vi "AlGaInPAs_Layer.vi"(2 "Debug Mode":bool, 3 "Elapsed Time (s)":dbl, 4 "State":enum16{"Edit", "Start", "Run", "End", "Idle"}(ring), 5 "Argument List In":string[](array[string])) -> (0 "Status Out":string, 1 "Argument List Out":string[](array[string]))   [LabVIEW 2011]
panel:
  out "Status Out 6":string
  out "Status Out 5":string
  out "Status Out 4":string
  out "Status Out 3":string
  out "In?":bool
  out "Ga?":bool
  out "Al?":bool
  out "AsH3?":bool
  out "PH3?":bool
  out "Status Out 2":string
  in  "AsH3 Flow":dbl
  in  "AsH3 run":bool
  in  "Al_run":bool
  in  "Al Flow":dbl
  in  "PH3 run":bool
  in  "In run":bool
  in  "Ga run":bool
  in  "PH3 Flow":dbl
  in  "In Flow":dbl
  in  "Ga Flow":dbl
  in  "Cancel":bool
  in  "OK":bool
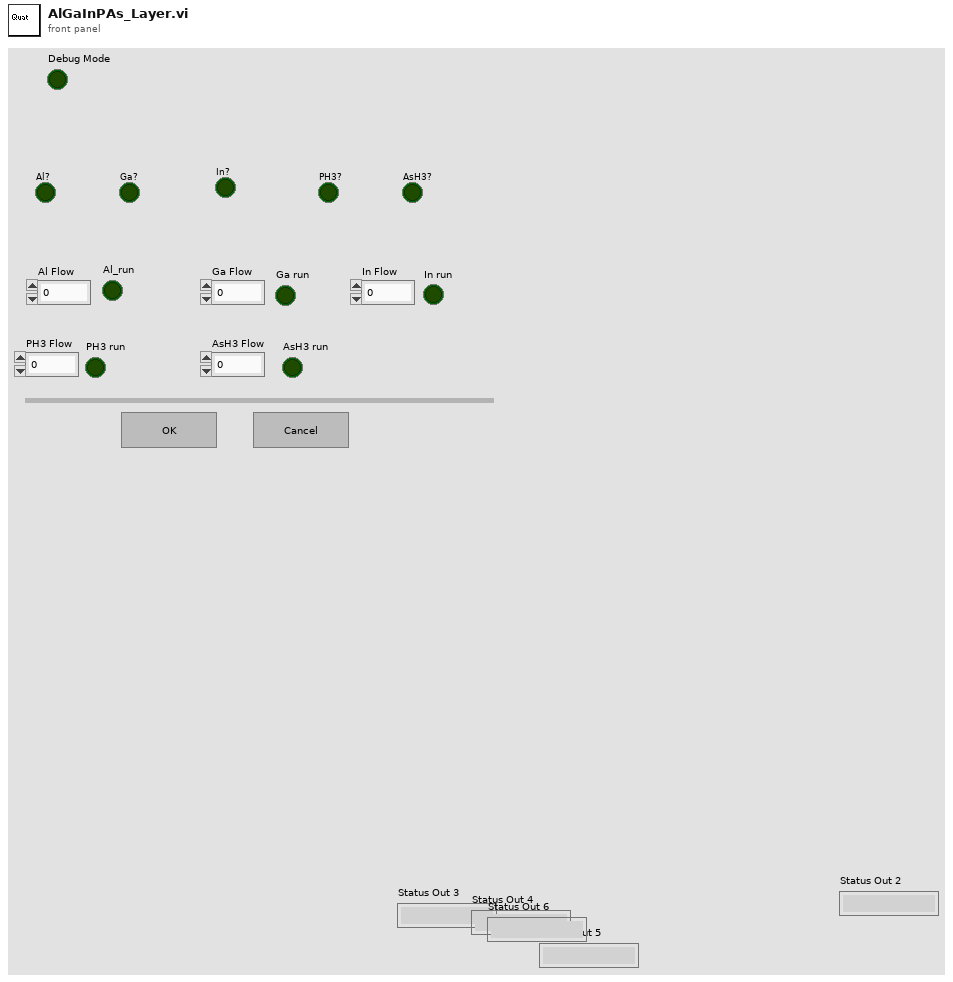
[diagram p1: front panel]
types:
  T1 = enum16{"Discrete", "Continuous", "Instantaneous"}
  T2 = enum32{"Invalid", "Default", "Floating", "Floating/Auto-Hide", "Modal"}
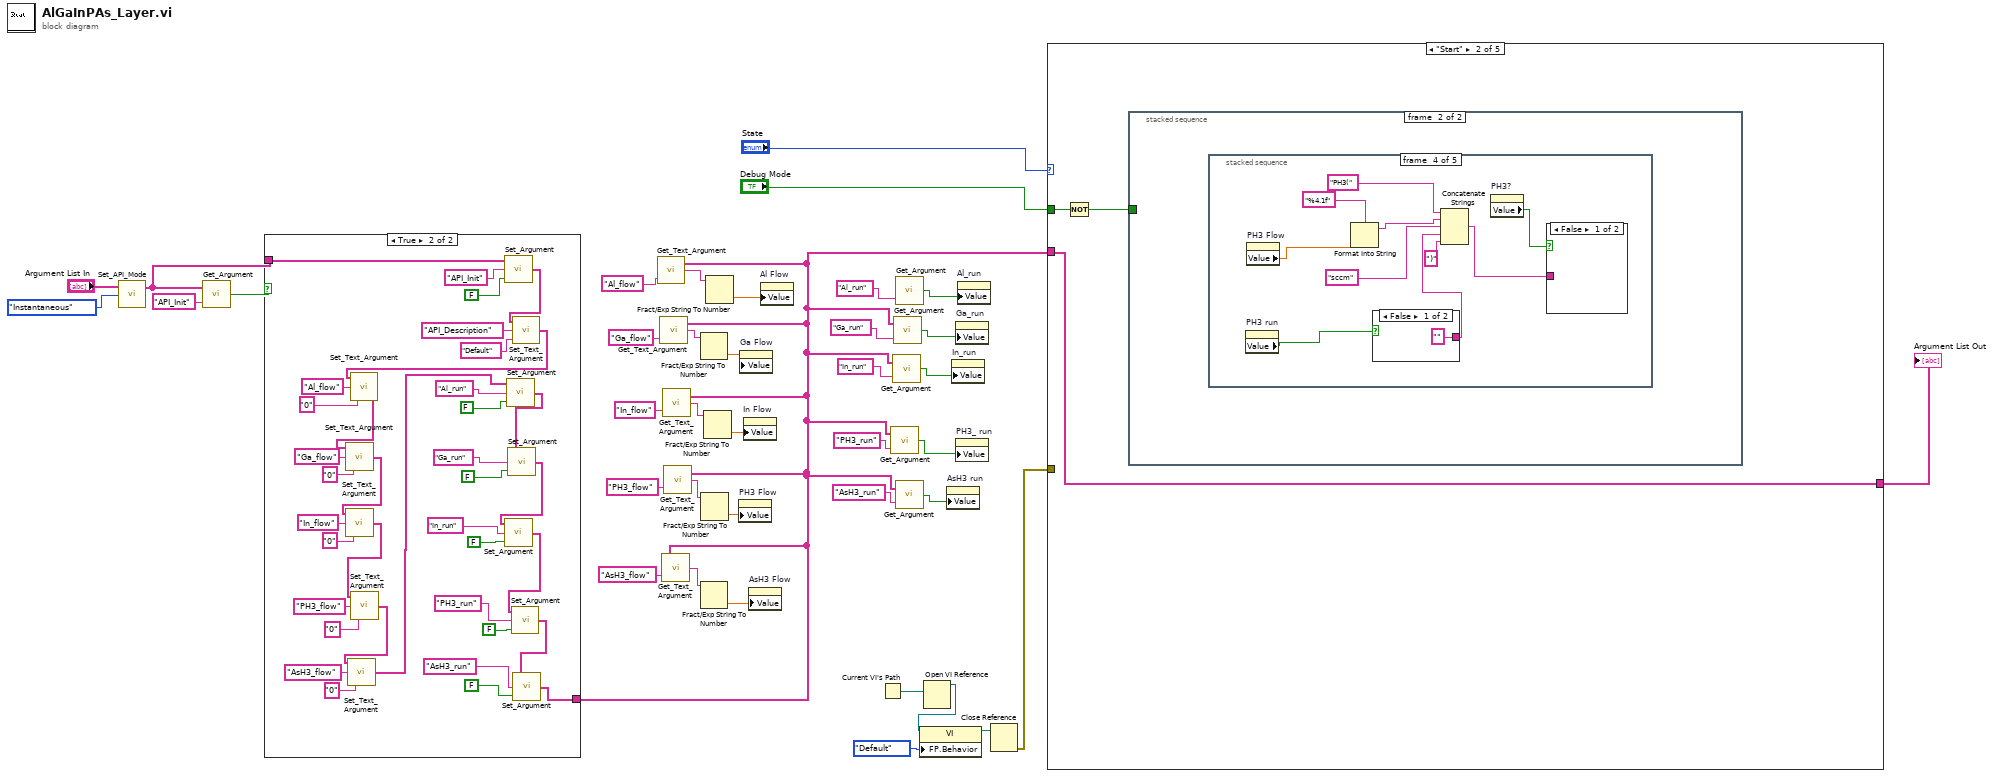
[diagram p0: block diagram]
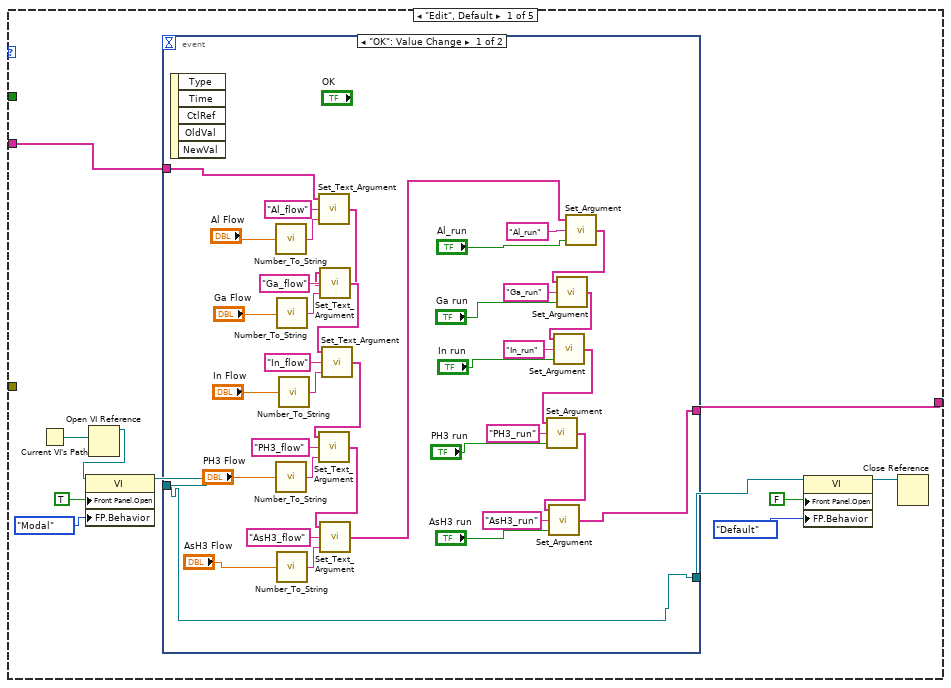
[diagram p3: hidden frame]
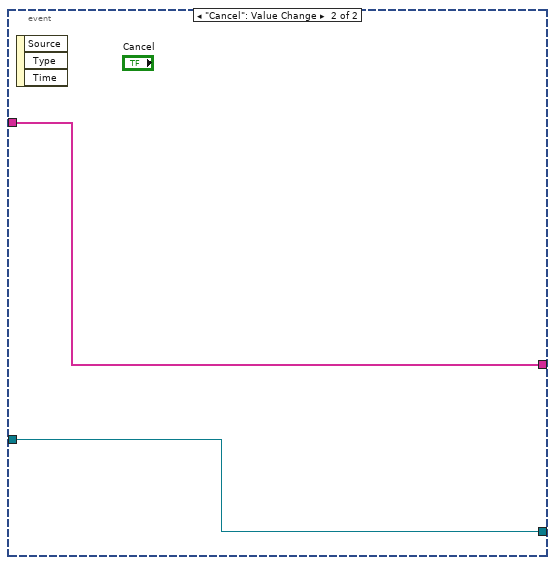
[diagram p4: hidden frame]
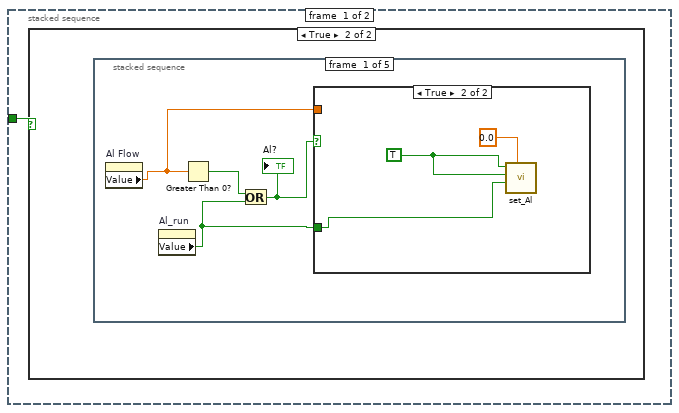
[diagram p5: hidden frame]
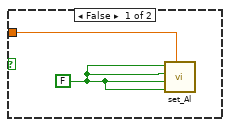
[diagram p7: hidden frame]
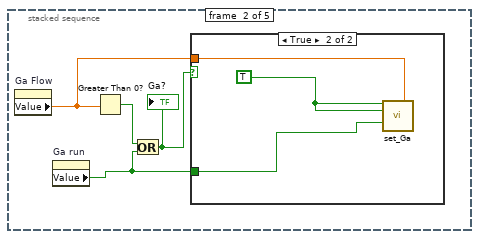
[diagram p8: hidden frame]
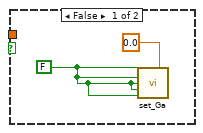
[diagram p9: hidden frame]
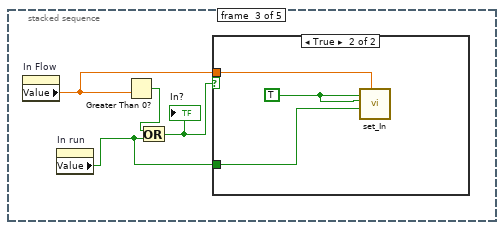
[diagram p10: hidden frame]
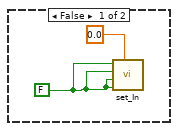
[diagram p11: hidden frame]
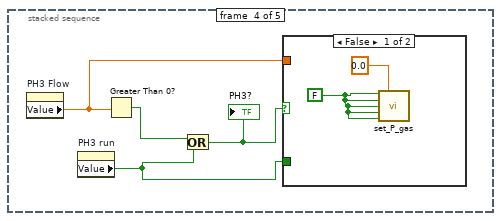
[diagram p12: hidden frame]
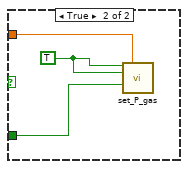
[diagram p13: hidden frame]
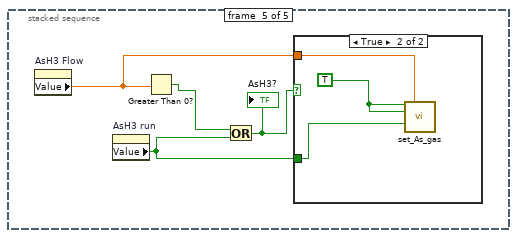
[diagram p14: hidden frame]
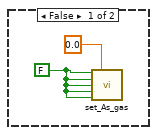
[diagram p15: hidden frame]
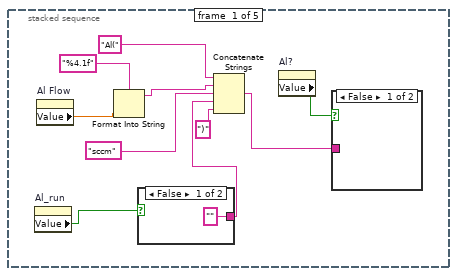
[diagram p16: hidden frame]
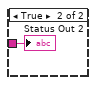
[diagram p17: hidden frame]
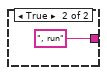
[diagram p18: hidden frame]
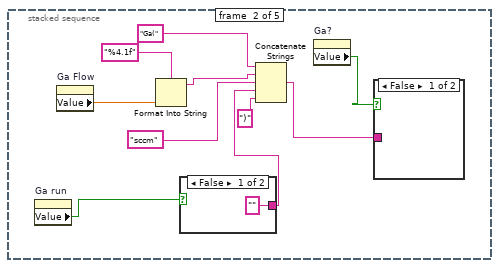
[diagram p19: hidden frame]
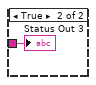
[diagram p20: hidden frame]
diagram:
  n1 = call "Set_API_Mode.vi"("API Mode"=T1."Instantaneous", "Argument List In"="Argument List In") -> ("Argument List Out"=w26:string[])  [unwired: 2 out]
  n2 = call "Get_Argument.vi"("Argument"="API_Init", "Argument List"=w26) -> ("Enabled"=w27:bool)
  n3 = case shown="True" w27 {
    tunnel: w26 -> [w40 w77]
    tunnel: [w40 w53] -> w5
    frame False {
    }
    frame True {
      n4 = call "Set_Argument.vi"("Enable"=FALSE, "Argument"="API_Init", "Argument List In"=w77) -> ("Argument List Out"=w74:string[])
      n5 = call "Set_Text_Argument.vi"("Text"="Default", "Argument"="API_Description", "Argument List In"=w74) -> ("Argument List Out"=w45:string[])
      n6 = call "Set_Text_Argument.vi"("Text"="0", "Argument"="Al_flow", "Argument List In"=w45) -> ("Argument List Out"=w44:string[])
      n7 = call "Set_Text_Argument.vi"("Text"="0", "Argument"="Ga_flow", "Argument List In"=w44) -> ("Argument List Out"=w67:string[])
      n8 = call "Set_Text_Argument.vi"("Text"="0", "Argument"="In_flow", "Argument List In"=w67) -> ("Argument List Out"=w43:string[])
      n9 = call "Set_Text_Argument.vi"("Text"="0", "Argument"="PH3_flow", "Argument List In"=w43) -> ("Argument List Out"=w55:string[])
      n10 = call "Set_Text_Argument.vi"("Text"="0", "Argument"="AsH3_flow", "Argument List In"=w55) -> ("Argument List Out"=w42:string[])
      n11 = call "Set_Argument.vi"("Enable"=FALSE, "Argument"="Al_run", "Argument List In"=w42) -> ("Argument List Out"=w48:string[])
      n12 = call "Set_Argument.vi"("Enable"=FALSE, "Argument"="Ga_run", "Argument List In"=w48) -> ("Argument List Out"=w58:string[])
      n13 = call "Set_Argument.vi"("Enable"=FALSE, "Argument"="In_run", "Argument List In"=w58) -> ("Argument List Out"=w41:string[])
      n14 = call "Set_Argument.vi"("Enable"=FALSE, "Argument"="PH3_run", "Argument List In"=w41) -> ("Argument List Out"=w51:string[])
      n15 = call "Set_Argument.vi"("Enable"=FALSE, "Argument"="AsH3_run", "Argument List In"=w51) -> ("Argument List Out"=w53:string[])
    }
  }
  n16 = call "Get_Text_Argument.vi"("Argument"="Al_flow", "Argument List"=w5) -> ("Text"=w6:string)
  n17 = call "Get_Text_Argument.vi"("Argument"="Ga_flow", "Argument List"=w5) -> ("Text"=w22:string)
  n18 = call "Get_Text_Argument.vi"("Argument"="AsH3_flow", "Argument List"=w5) -> ("Text"=w18:string)
  n19 = call "Get_Text_Argument.vi"("Argument"="In_flow", "Argument List"=w5) -> ("Text"=w20:string)
  n20 = call "Get_Text_Argument.vi"("Argument"="PH3_flow", "Argument List"=w5) -> ("Text"=w17:string)
  n21 = Fract/Exp String To Number(string=w22) -> (number=w21:dbl)  [unwired: 4 out]
  n22 = Fract/Exp String To Number(string=w18) -> (number=w1:dbl)  [unwired: 4 out]
  n23 = Fract/Exp String To Number(string=w17) -> (number=w16:dbl)  [unwired: 4 out]
  n24 = Fract/Exp String To Number(string=w20) -> (number=w19:dbl)  [unwired: 4 out]
  n25 = Fract/Exp String To Number(string=w6) -> (number=w2:dbl)  [unwired: 4 out]
  n26 = property on="PH3 Flow" class="DigNum (strict)"("Value"=w16) -> ()  [unwired: 2 in, 2 out]
  n27 = property on="Ga Flow" class="DigNum (strict)"("Value"=w21) -> ()  [unwired: 2 in, 2 out]
  n28 = property on="In Flow" class="DigNum (strict)"("Value"=w19) -> ()  [unwired: 2 in, 2 out]
  n29 = property on="AsH3 Flow" class="DigNum (strict)"("Value"=w1) -> ()  [unwired: 2 in, 2 out]
  n30 = property on="Al Flow" class="DigNum (strict)"("Value"=w2) -> ()  [unwired: 2 in, 2 out]
  n31 = Current VI's Path() -> (path=w35:path)
  n32 = call "Get_Argument.vi"("Argument"="PH3_run", "Argument List"=w5) -> ("Enabled"=w12:bool)
  n33 = call "Get_Argument.vi"("Argument"="In_run", "Argument List"=w5) -> ("Enabled"=w13:bool)
  n34 = call "Get_Argument.vi"("Argument"="Ga_run", "Argument List"=w5) -> ("Enabled"=w14:bool)
  n35 = call "Get_Argument.vi"("Argument"="Al_run") -> ("Enabled"=w4:bool)  [unwired: 1 in]
  n36 = call "Get_Argument.vi"("Argument"="AsH3_run", "Argument List"=w5) -> ("Enabled"=w3:bool)
  n37 = Open VI Reference(vi path=w35) -> (vi reference=w34:refnum<vi>)  [unwired: 1 in, 5 out]
  n38 = property class="VI"(reference=w34, "FP.Behavior"=T2."Default" ("Front Panel Window:Behavior")) -> (reference out=w32:refnum<vi>)  [unwired: 1 in, 1 out]
  n39 = property on="AsH3 run" class="Bool (strict)"("Value"=w3) -> ()  [unwired: 2 in, 2 out]
  n40 = property on="In_run" class="Bool (strict)"("Value"=w13) -> ()  [unwired: 2 in, 2 out]
  n41 = property on="Ga_run" class="Bool (strict)"("Value"=w14) -> ()  [unwired: 2 in, 2 out]
  n42 = property on="PH3_ run" class="Bool (strict)"("Value"=w12) -> ()  [unwired: 2 in, 2 out]
  n43 = property on="Al_run" class="Bool (strict)"("Value"=w4) -> ()  [unwired: 2 in, 2 out]
  n44 = Close Reference(reference=w32) -> (error out=w31:errorcluster)  [unwired: 1 in]
  n45 = case shown="\"Start\"" "State" {
    tunnel: [w88 w130 w242 w247 w248] -> w38
    tunnel: w5 -> [w87 w130 w242 w247 w248]
    tunnel: "Debug Mode" -> [_ w129 _ _ _]
    tunnel: w31 -> [_ _ _ _ _]
    frame "Edit", Default {
      n46 = Current VI's Path() -> (path=w82:path)
      n47 = Open VI Reference(vi path=w82) -> (vi reference=w81:refnum<vi>)  [unwired: 1 in, 5 out]
      n48 = property class="VI"(reference=w81, "Front Panel.Open"=TRUE ("Front Panel Window:Open"), "FP.Behavior"=T2."Modal" ("Front Panel Window:Behavior")) -> (reference out=w85:refnum<vi>)  [unwired: 1 in, 1 out]
      n49 = event shown="[0] \"OK\": Value Change" {
        selector: _ -> [_ _]
        dyn-events: _ -> [_ _]
        timeout: _ -> [_ _]
        tunnel: w87 -> [w98 w126]
        tunnel: [w105 w126] -> w88
        tunnel: [w89 w127] -> w84
        tunnel: w85 -> [w89 w127]
        event "OK": Value Change {
          n50 = event-data() -> ()  [unwired: 6 out]
          n51 = call "Number_To_String.vi"("Number"="Al Flow") -> ("String"=w99:string)
          n52 = call "Number_To_String.vi"("Number"="PH3 Flow") -> ("String"=w117:string)
          n53 = call "Number_To_String.vi"("Number"="Ga Flow") -> ("String"=w124:string)
          n54 = call "Number_To_String.vi"("Number"="AsH3 Flow") -> ("String"=w95:string)
          n55 = call "Number_To_String.vi"("Number"="In Flow") -> ("String"=w121:string)
          n56 = call "Set_Text_Argument.vi"("Text"=w99, "Argument"="Al_flow", "Argument List In"=w98) -> ("Argument List Out"=w97:string[])
          n57 = call "Set_Text_Argument.vi"("Text"=w124, "Argument"="Ga_flow", "Argument List In"=w97) -> ("Argument List Out"=w120:string[])
          n58 = call "Set_Text_Argument.vi"("Text"=w121, "Argument"="In_flow", "Argument List In"=w120) -> ("Argument List Out"=w92:string[])
          n59 = call "Set_Text_Argument.vi"("Text"=w117, "Argument"="PH3_flow", "Argument List In"=w92) -> ("Argument List Out"=w93:string[])
          n60 = call "Set_Text_Argument.vi"("Text"=w95, "Argument"="AsH3_flow", "Argument List In"=w93) -> ("Argument List Out"=w94:string[])
          n61 = call "Set_Argument.vi"("Enable"="Al_run", "Argument"="Al_run", "Argument List In"=w94) -> ("Argument List Out"=w91:string[])
          n62 = call "Set_Argument.vi"("Enable"="Ga run", "Argument"="Ga_run", "Argument List In"=w91) -> ("Argument List Out"=w109:string[])
          n63 = call "Set_Argument.vi"("Enable"="In run", "Argument"="In_run", "Argument List In"=w109) -> ("Argument List Out"=w103:string[])
          n64 = call "Set_Argument.vi"("Enable"="PH3 run", "Argument"="PH3_run", "Argument List In"=w103) -> ("Argument List Out"=w104:string[])
          n65 = call "Set_Argument.vi"("Enable"="AsH3 run", "Argument"="AsH3_run", "Argument List In"=w104) -> ("Argument List Out"=w105:string[])
        }
        event "Cancel": Value Change {
          n66 = event-data() -> ()  [unwired: 4 out]
        }
      }
      n67 = property class="VI"(reference=w84, "Front Panel.Open"=FALSE ("Front Panel Window:Open"), "FP.Behavior"=T2."Default" ("Front Panel Window:Behavior")) -> (reference out=w78:refnum<vi>)  [unwired: 1 in, 1 out]
      n68 = Close Reference(reference=w78) -> ()  [unwired: 1 in, 1 out]
    }
    frame "Start" {
      n69 = Not(x=w129) -> (.not. x?=w128:bool)
      n70 = stacked-sequence {
        tunnel: w128 -> [w131 _]
        frame #0 {
          n71 = case shown="True" w131 {
            frame False {
            }
            frame True {
              n72 = stacked-sequence {
                frame #0 {
                  n73 = property on="Al Flow" class="DigNum (strict)"() -> ("Value"=w135:dbl)  [unwired: 2 in, 2 out]
                  n74 = property on="Al_run" class="Bool (strict)"() -> ("Value"=w132:bool)  [unwired: 2 in, 2 out]
                  n75 = Greater Than 0?(x=w135) -> (x > 0?=w134:bool)
                  n76 = Or(x=w134, y=w132) -> (x .or. y?=w133:bool)
                  "Al?" <- w133
                  n77 = case shown="True" w133 {
                    tunnel: w135 -> [w137 _]
                    tunnel: w132 -> [_ w138]
                    frame False {
                      w136 = FALSE ("Al Active")
                      n78 = call "set_Al.vi"("Aluminum Flow"=w137, "Al Remote"=w136, "Al Run"=w136, "Al Bubbler"=w136, "Al Active"=w136) -> ()  [unwired: 5 out]
                    }
                    frame True {
                      w139 = TRUE ("Al Active")
                      n79 = call "set_Al.vi"("Aluminum Flow"=0.0, "Al Run"=w138, "Al Bubbler"=w139, "Al Active"=w139) -> ()  [unwired: 1 in, 5 out]
                    }
                  }
                }
                frame #1 {
                  n80 = property on="Ga Flow" class="DigNum (strict)"() -> ("Value"=w144:dbl)  [unwired: 2 in, 2 out]
                  n81 = property on="Ga run" class="Bool (strict)"() -> ("Value"=w141:bool)  [unwired: 2 in, 2 out]
                  n82 = Greater Than 0?(x=w144) -> (x > 0?=w143:bool)
                  n83 = Or(x=w143, y=w141) -> (x .or. y?=w142:bool)
                  "Ga?" <- w142
                  n84 = case shown="True" w142 {
                    tunnel: w144 -> [_ w149]
                    tunnel: w141 -> [_ w147]
                    frame False {
                      w145 = FALSE ("Ga Active")
                      n85 = call "set_Ga.vi"("Ga Active"=w145, "Ga Flow 1"=0.0, "Ga Bubbler"=w145, "Ga H2 Dilute"=w145, "Ga Run"=w145, "Ga Remote"=w145) -> ()  [unwired: 2 in, 8 out]
                    }
                    frame True {
                      w148 = TRUE ("Ga Active")
                      n86 = call "set_Ga.vi"("Ga Active"=w148, "Ga Flow 1"=w149, "Ga Bubbler"=w148, "Ga Run"=w147) -> ()  [unwired: 4 in, 8 out]
                    }
                  }
                }
                frame #2 {
                  n87 = property on="In Flow" class="DigNum (strict)"() -> ("Value"=w153:dbl)  [unwired: 2 in, 2 out]
                  n88 = property on="In run" class="Bool (strict)"() -> ("Value"=w150:bool)  [unwired: 2 in, 2 out]
                  n89 = Greater Than 0?(x=w153) -> (x > 0?=w152:bool)
                  n90 = Or(x=w152, y=w150) -> (x .or. y?=w151:bool)
                  "In?" <- w151
                  n91 = case shown="True" w151 {
                    tunnel: w153 -> [_ w158]
                    tunnel: w150 -> [_ w156]
                    frame False {
                      w155 = FALSE ("In Remote")
                      n92 = call "set_In.vi"("Indium Flow"=0.0, "In Remote"=w155, "In Run"=w155, "In Bubbler"=w155, "In Active"=w155) -> ()  [unwired: 5 out]
                    }
                    frame True {
                      w157 = TRUE ("In Run")
                      n93 = call "set_In.vi"("Indium Flow"=w158, "In Run"=w156, "In Bubbler"=w157, "In Active"=w157) -> ()  [unwired: 1 in, 5 out]
                    }
                  }
                }
                frame #3 {
                  n94 = property on="PH3 Flow" class="DigNum (strict)"() -> ("Value"=w162:dbl)  [unwired: 2 in, 2 out]
                  n95 = property on="PH3 run" class="Bool (strict)"() -> ("Value"=w159:bool)  [unwired: 2 in, 2 out]
                  n96 = Greater Than 0?(x=w162) -> (x > 0?=w161:bool)
                  n97 = Or(x=w161, y=w159) -> (x .or. y?=w160:bool)
                  "PH3?" <- w160
                  n98 = case shown="False" w160 {
                    tunnel: w162 -> [_ w167]
                    tunnel: w159 -> [_ w165]
                    frame False {
                      w163 = FALSE ("P_Gas Active")
                      n99 = call "set_P_gas.vi"("P_Gas Active"=w163, "P_Gas Flow"=0.0, "P_Gas In"=w163, "P_Gas H2 In"=w163, "P_Gas Run"=w163, "P_Gas Remote"=w163) -> ()  [unwired: 10 out]
                    }
                    frame True {
                      w166 = TRUE ("P_Gas Active")
                      n100 = call "set_P_gas.vi"("P_Gas Active"=w166, "P_Gas Flow"=w167, "P_Gas In"=w166, "P_Gas Run"=w165) -> ()  [unwired: 2 in, 10 out]
                    }
                  }
                }
                frame #4 {
                  n101 = property on="AsH3 Flow" class="DigNum (strict)"() -> ("Value"=w171:dbl)  [unwired: 2 in, 2 out]
                  n102 = property on="AsH3 run" class="Bool (strict)"() -> ("Value"=w168:bool)  [unwired: 2 in, 2 out]
                  n103 = Greater Than 0?(x=w171) -> (x > 0?=w170:bool)
                  n104 = Or(x=w170, y=w168) -> (x .or. y?=w169:bool)
                  "AsH3?" <- w169
                  n105 = case shown="True" w169 {
                    tunnel: w171 -> [_ w176]
                    tunnel: w168 -> [_ w174]
                    frame False {
                      w172 = FALSE ("As_Gas Active")
                      n106 = call "set_As_gas.vi"("As_Gas Active"=w172, "As_Gas Flow"=0.0, "As_Gas In"=w172, "As_Gas H2"=w172, "As_Gas Run"=w172, "As_Gas Remote"=w172) -> ()  [unwired: 10 out]
                    }
                    frame True {
                      w175 = TRUE ("As_Gas Active")
                      n107 = call "set_As_gas.vi"("As_Gas Active"=w175, "As_Gas Flow"=w176, "As_Gas In"=w175, "As_Gas Run"=w174) -> ()  [unwired: 2 in, 10 out]
                    }
                  }
                }
              }
            }
          }
        }
        frame #1 {
          n108 = stacked-sequence {
            frame #0 {
              n109 = property on="Al_run" class="Bool (strict)"() -> ("Value"=w184:bool)  [unwired: 2 in, 2 out]
              n110 = property on="Al Flow" class="DigNum (strict)"() -> ("Value"=w179:dbl)  [unwired: 2 in, 2 out]
              n111 = Format Into String(format string="%4.1f", w179) -> (resulting string=w178:string)  [unwired: 2 in, 1 out]
              n112 = case shown="False" w184 {
                tunnel: ["" ", run"] -> w183
                frame False {
                }
                frame True {
                }
              }
              n113 = Concatenate Strings("Al(" ("string"), w178, "sccm" ("string"), w183, ")" ("string")) -> (w180:string)
              n114 = property on="Al?" class="Bool (strict)"() -> ("Value"=w181:bool)  [unwired: 2 in, 2 out]
              n115 = case shown="False" w181 {
                tunnel: w180 -> [_ w187]
                frame False {
                }
                frame True {
                  "Status Out 2" <- w187
                }
              }
            }
            frame #1 {
              n116 = property on="Ga run" class="Bool (strict)"() -> ("Value"=w191:bool)  [unwired: 2 in, 2 out]
              n117 = property on="Ga Flow" class="DigNum (strict)"() -> ("Value"=w192:dbl)  [unwired: 2 in, 2 out]
              n118 = Format Into String(format string="%4.1f", w192) -> (resulting string=w194:string)  [unwired: 2 in, 1 out]
              n119 = case shown="False" w191 {
                tunnel: ["" ", run"] -> w197
                frame False {
                }
                frame True {
                }
              }
              n120 = Concatenate Strings("Ga(" ("string"), w194, "sccm" ("string"), w197, ")" ("string")) -> (w195:string)
              n121 = property on="Ga?" class="Bool (strict)"() -> ("Value"=w190:bool)  [unwired: 2 in, 2 out]
              n122 = case shown="False" w190 {
                tunnel: w195 -> [_ w200]
                frame False {
                }
                frame True {
                  "Status Out 3" <- w200
                }
              }
            }
            frame #2 {
              n123 = property on="In run" class="Bool (strict)"() -> ("Value"=w204:bool)  [unwired: 2 in, 2 out]
              n124 = property on="In Flow" class="DigNum (strict)"() -> ("Value"=w205:dbl)  [unwired: 2 in, 2 out]
              n125 = Format Into String(format string="%4.1f", w205) -> (resulting string=w207:string)  [unwired: 2 in, 1 out]
              n126 = case shown="False" w204 {
                tunnel: ["" ", run"] -> w210
                frame False {
                }
                frame True {
                }
              }
              n127 = Concatenate Strings("In(" ("string"), w207, "sccm" ("string"), w210, ")" ("string")) -> (w208:string)
              n128 = property on="In?" class="Bool (strict)"() -> ("Value"=w203:bool)  [unwired: 2 in, 2 out]
              n129 = case shown="False" w203 {
                tunnel: w208 -> [_ w213]
                frame False {
                }
                frame True {
                  "Status Out 4" <- w213
                }
              }
            }
            frame #3 {
              n130 = property on="PH3 run" class="Bool (strict)"() -> ("Value"=w216:bool)  [unwired: 2 in, 2 out]
              n131 = property on="PH3 Flow" class="DigNum (strict)"() -> ("Value"=w217:dbl)  [unwired: 2 in, 2 out]
              n132 = Format Into String(format string="%4.1f", w217) -> (resulting string=w220:string)  [unwired: 2 in, 1 out]
              n133 = case shown="False" w216 {
                tunnel: ["" ", run"] -> w223
                frame False {
                }
                frame True {
                }
              }
              n134 = Concatenate Strings("PH3(" ("string"), w220, "sccm" ("string"), w223, ")" ("string")) -> (w221:string)
              n135 = property on="PH3?" class="Bool (strict)"() -> ("Value"=w218:bool)  [unwired: 2 in, 2 out]
              n136 = case shown="False" w218 {
                tunnel: w221 -> [_ w226]
                frame False {
                }
                frame True {
                  "Status Out 5" <- w226
                }
              }
            }
            frame #4 {
              n137 = property on="AsH3 run" class="Bool (strict)"() -> ("Value"=w230:bool)  [unwired: 2 in, 2 out]
              n138 = property on="AsH3 Flow" class="DigNum (strict)"() -> ("Value"=w231:dbl)  [unwired: 2 in, 2 out]
              n139 = Format Into String(format string="%4.2f", w231) -> (resulting string=w233:string)  [unwired: 2 in, 1 out]
              n140 = case shown="False" w230 {
                tunnel: ["" ", run"] -> w236
                frame False {
                }
                frame True {
                }
              }
              n141 = Concatenate Strings("Al(" ("string"), w233, "sccm" ("string"), w236, ")" ("string")) -> (w234:string)
              n142 = property on="AsH3?" class="Bool (strict)"() -> ("Value"=w229:bool)  [unwired: 2 in, 2 out]
              n143 = case shown="False" w229 {
                tunnel: w234 -> [_ w239]
                frame False {
                }
                frame True {
                  "Status Out 6" <- w239
                }
              }
            }
          }
        }
      }
    }
    frame "Run" {
      n144 = call "Seconds_To_String.vi"("Seconds"="Elapsed Time (s)") -> ("Output String"=w244:string)
      n145 = Concatenate Strings("Elapsed time: " ("string"), w244) -> (→"Status Out":string)
    }
    frame "End" {
    }
    frame "Idle" {
    }
  }
  "Argument List Out" <- w38
